vi "Write VI Information Changed Msg.vi"(10 "Interface.lvlib:VI Information Changed Msg.lvclass":refnum<class "VI Information Changed Msg.lvclass">, 11 "Interface in":refnum<class "Interface.lvclass">) -> (3 "Interface out":refnum<class "Interface.lvclass">)   [LabVIEW 2018, in "Interface.lvlib" / "Interface.lvclass"]
uses:
  Interface.lvclass
  Interface Messages/VI Information Changed Msg/VI Information Changed Msg.lvclass
  Interface.lvclass/Interface.ctl
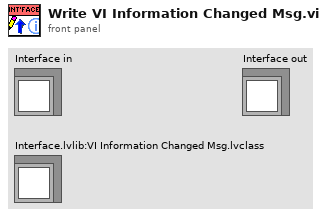
[diagram p1: front panel]
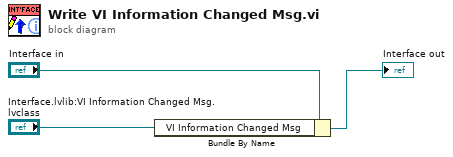
[diagram p0: block diagram]
diagram:
  n1 = Bundle By Name(cluster="Interface in", "VI Information Changed Msg"="Interface.lvlib:VI Information Changed Msg.lvclass") -> (→"Interface out":refnum<class "Interface.lvclass">)
